vi "XY Moving Median.vi"(9 "Y Array":dbl[](array[numeric]), 10 "Moving Median":dbl, 11 "X Array":dbl[](array[numeric])) -> (0 "Small Final Median?":bool, 2 "Y Array":dbl[](array[numeric]), 3 "X Array":dbl[](array[numeric]))   [LabVIEW 2023]
uses:
  e787c073-bad0-ad4f-bba6-7e6257a1fe3c.vi
  <vilib>/Array/Sort 2D Array - Pop Stack.vi
  <vilib>/Array/Sort 2D Array - Push Stack.vi
  e787c073-bad0-ad4f-bba6-7e6257a1fe3c.vi/269d4b3b-47f5-49e3-8884-44851e4dd9d5.vi
  e787c073-bad0-ad4f-bba6-7e6257a1fe3c.vi/6d99389c-673d-4efb-bf33-19b32bcf4cf8.vi
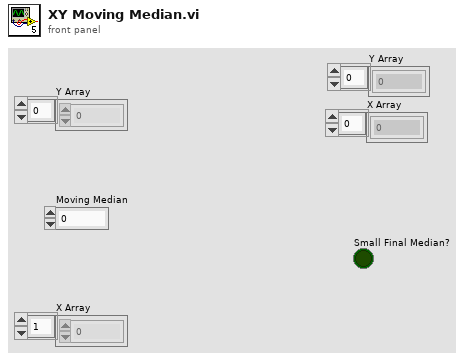
[diagram p1: front panel]
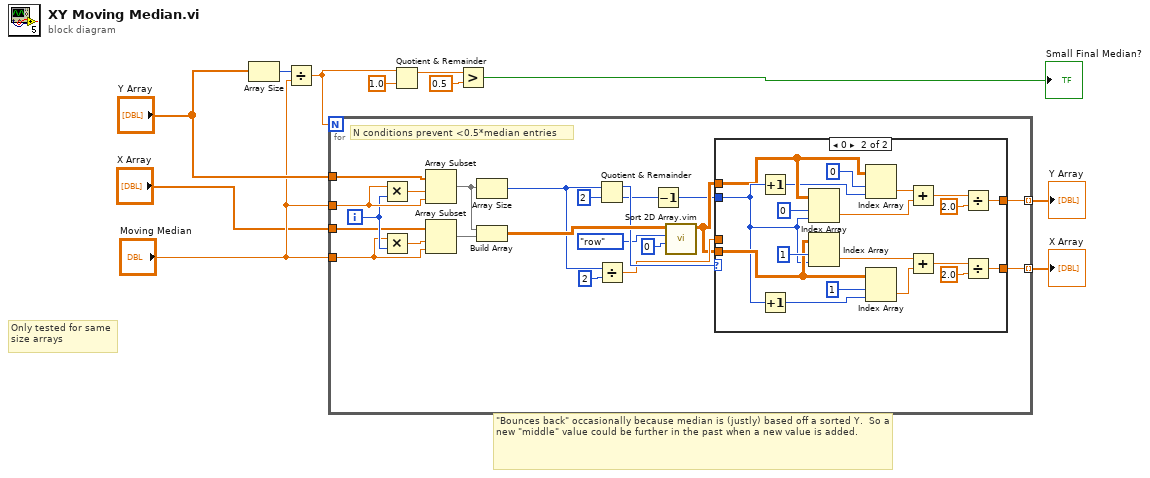
[diagram p0: block diagram]
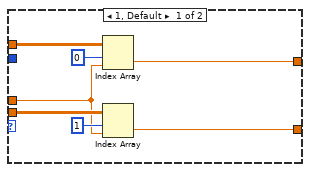
[diagram p2: hidden frame]
diagram:
  # "\"Bounces back\" occasionally because median is (justly) based off a sorted Y.  So a new \"middle\" value could be further in the past when a new value is added."
  # "Only tested for same size arrays"
  n1 = Array Size(array="Y Array") -> (size(s)=w9:i32)
  n2 = Divide(x=w9, y="Moving Median") -> (x/y=w7:dbl)
  n3 = for {
    N: w7 -> [_]
    tunnel: "Moving Median" -> [w33]
    tunnel: "Y Array" -> [w32]
    tunnel: [w16] -> w11 mode=indexing
    tunnel: "Moving Median" -> [w28]
    tunnel: "X Array" -> [w27]
    tunnel: [w15] -> w1 mode=indexing
    i -> [w30]
    # "N conditions prevent <0.5*median entries"
    n4 = Multiply(x=w33, y=w30) -> (x*y=w31:dbl)
    n5 = Multiply(x=w28, y=w30) -> (x*y=w29:dbl)
    n6 = Array Subset(array=w32, index=w31, length=w33) -> (w23:dbl[])
    n7 = Array Subset(array=w27, index=w29, length=w28) -> (w26:dbl[])
    n8 = Array Size(array=w23) -> (size(s)=w20:i32)
    n9 = Build Array(w23, w26) -> (w25:dbl[][])
    n10 = Quotient & Remainder(x=w20, y=2) -> (x-y*floor(x/y)=w21:i32, floor(x/y)=w14:i32)
    n11 = Divide(x=w20, y=2) -> (x/y=w18:dbl)
    n12 = Decrement(x=w14) -> (x-1=w12:i32)
    n13 = call "Sort 2D Array.vim"("index"=0, "dimension to index (column)"=enum16{"column", "row"}."row", "2D array"=w25) -> ("sorted 2D array"=w17:dbl[][])  [unwired: 7 in, 1 out]
    n14 = case shown="0" w21 {
      tunnel: w17 -> [w38 w56]
      tunnel: w18 -> [w36 _]
      tunnel: w17 -> [w37 w47]
      tunnel: [w35 w41] -> w16
      tunnel: [w34 w50] -> w15
      tunnel: w12 -> [_ w48]
      frame 1, Default {
        n15 = Index Array(array=w37, index (row)=0 ("index"), index (col)=w36) -> (element=w35:dbl)
        n16 = Index Array(array=w38, index (row)=1 ("index"), index (col)=w36) -> (element=w34:dbl)
      }
      frame 0 {
        n17 = Increment(x=w48) -> (x+1=w46:i32)
        n18 = Increment(x=w48) -> (x+1=w55:i32)
        n19 = Index Array(array=w47, index (row)=0, index (col)=w48) -> (element=w42:dbl)
        n20 = Index Array(array=w56, index (row)=1, index (col)=w48) -> (element=w54:dbl)
        n21 = Index Array(array=w47, index (row)=0, index (col)=w46) -> (element=w43:dbl)
        n22 = Index Array(array=w56, index (row)=1, index (col)=w55) -> (element=w53:dbl)
        n23 = Add(x=w43, y=w42) -> (x+y=w45:dbl)
        n24 = Add(x=w54, y=w53) -> (x+y=w52:dbl)
        n25 = Divide(x=w45, y=2.0) -> (x/y=w41:dbl)
        n26 = Divide(x=w52, y=2.0) -> (x/y=w50:dbl)
      }
    }
  }
  "Y Array" <- w11
  "X Array" <- w1
  n27 = Quotient & Remainder(x=w7, y=1.0) -> (x-y*floor(x/y)=w5:dbl)  [unwired: 1 out]
  n28 = Greater?(x=w5, y=0.5) -> (0:→"Small Final Median?":bool)
